vi "RampRateMultiple.vi"(6 "return immediately":bool, 7 "ramp rates":dbl[](array[numeric]), 8 "error in (no error)":T1, 9 "task id":i32(ring) items=["TLibrary", "T01", "T02", "T03", "T04", "T05", "T06", "T07", "T08", "T09", "T10", "T11", "T12", "T13", "T14", "T15", "T16", "T17", "T18", "T19", "T20", "T21", "T22", "T23", "T24", "T25", "T26", "T27", "T28", "T29", "T30", "T31"], 10 "axis names":string[](array[string]), 11 "controller in":refnum<k24>) -> (0 "error out (no error)":T1, 3 "controller out":refnum<k24>)   [LabVIEW 2020, in "Aerotech.lvlib"]
doc: "Ramp rate sets the acceleration and deceleration rates for its respective axis name."
uses:
  Aerotech.lvlib
  C:/Users/HEP/Documents/GitHub/UCSB-Gantry-HEP/Drivers/Aerotech A3200/Bin/Aerotech.A3200.LabVIEW.dll
  UCSB-Gantry-HEP/Drivers/Aerotech A3200/Bin/Aerotech.A3200.LabVIEW.dll
  C:/Program Files (x86)/Aerotech/A3200/LabVIEW/2010/Bin/Aerotech.A3200.dll
  Program Files (x86)/Aerotech/A3200/LabVIEW/2010/Bin/Aerotech.A3200.dll
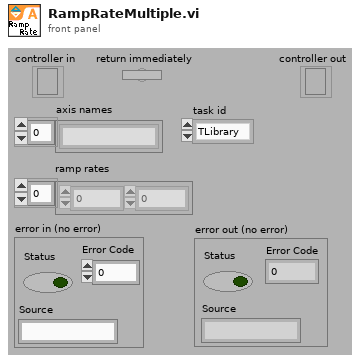
[diagram p1: front panel]
types:
  T1 = cluster{"Status":bool, "Error Code":i32, "Source":string}
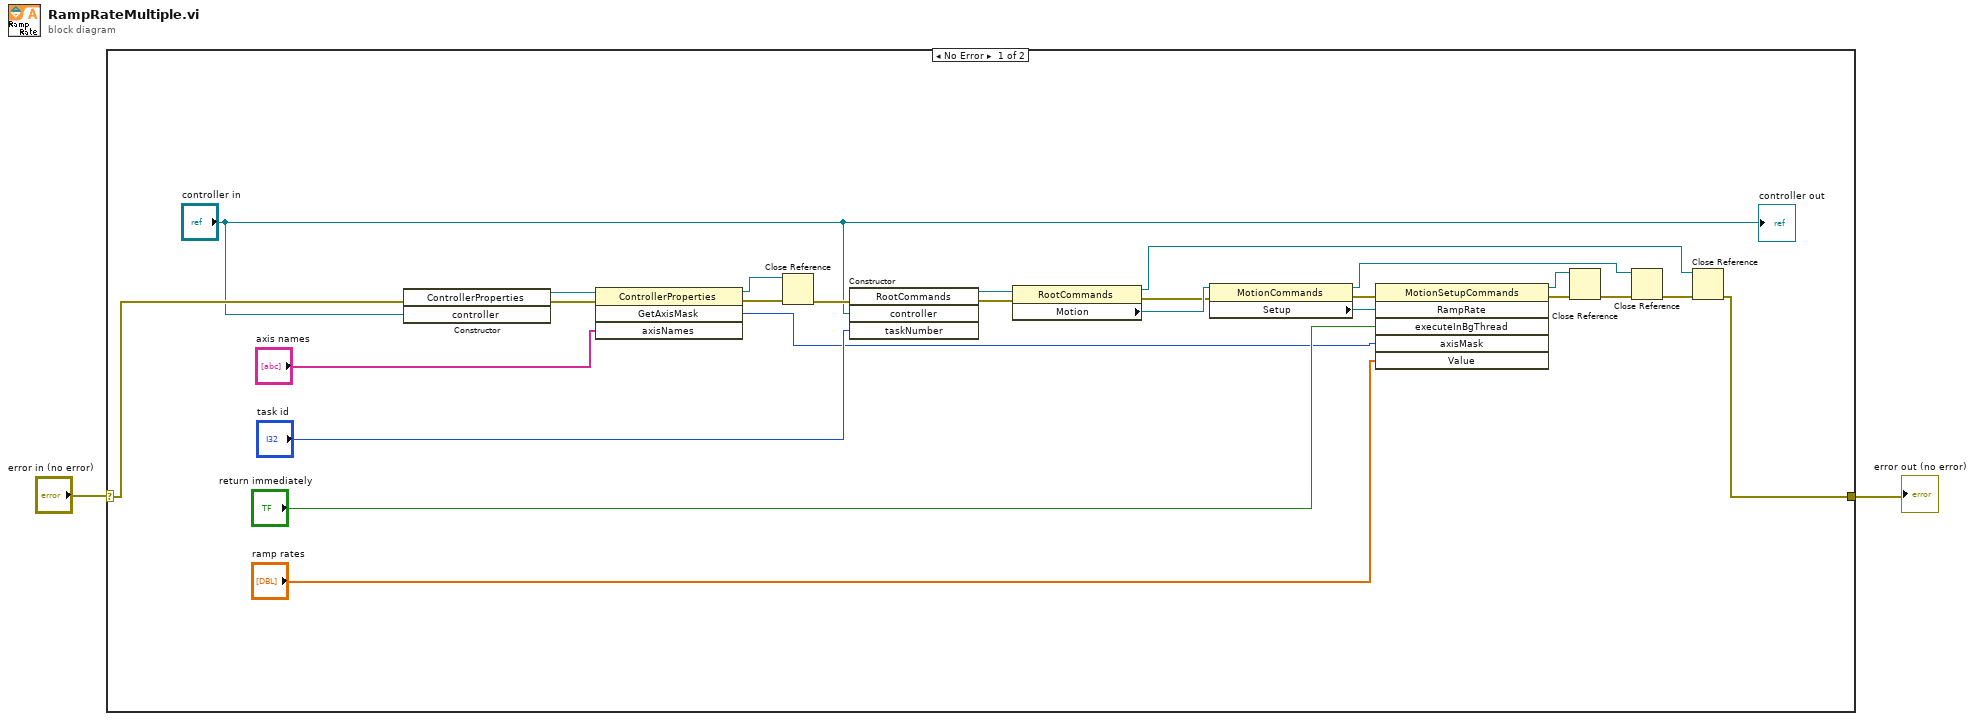
[diagram p0: block diagram]
diagram:
  n1 = case shown="No Error" "error in (no error)" {
    selector: "error in (no error)" -> [w21 w28]
    tunnel: [w5 w28] -> w1
    frame No Error {
      n2 = constructor class="ControllerProperties"(error in=w21, "controller"="controller in") -> (reference out=w27:refnum<k24>, error out=w26:errorcluster)  [unwired: 2 in, 2 out]
      n3 = invoke class="ControllerProperties" method="GetAxisMask"(reference=w27, error in=w26, "axisNames"="axis names") -> (reference out=w23:refnum<k24>, error out=w24:errorcluster, "GetAxisMask"=w12:i32)  [unwired: 1 in, 1 out]
      n4 = Close Reference(reference=w23, error in (no error)=w24) -> (error out=w22:errorcluster)
      n5 = constructor class="RootCommands"(error in=w22, "controller"="controller in", "taskNumber"="task id") -> (reference out=w18:refnum<k24>, error out=w19:errorcluster)  [unwired: 2 in, 3 out]
      n6 = property class="RootCommands"(reference=w18, error in=w19) -> (reference out=w6:refnum<k24>, error out=w16:errorcluster, "Motion"=w17:refnum<k24>)
      n7 = property class="MotionCommands"(reference=w17, error in=w16) -> (reference out=w7:refnum<k24>, error out=w15:errorcluster, "Setup"=w14:refnum<k24>)
      n8 = invoke class="MotionSetupCommands" method="RampRate"(reference=w14, error in=w15, "executeInBgThread"="return immediately", "axisMask"=w12, "Value"="ramp rates") -> (reference out=w10:refnum<k24>, error out=w11:errorcluster)  [unwired: 1 in, 4 out]
      n9 = Close Reference(reference=w10, error in (no error)=w11) -> (error out=w9:errorcluster)
      n10 = Close Reference(reference=w7, error in (no error)=w9) -> (error out=w8:errorcluster)
      n11 = Close Reference(reference=w6, error in (no error)=w8) -> (error out=w5:errorcluster)
      "controller out" <- "controller in"
    }
    frame Error {
    }
  }
  "error out (no error)" <- w1
